vi "HPRF File Producer.vi"(3 "Source File":path=path "C:/ScopeBinaryData.bin", 4 "error in (no error)":errorcluster, 5 "# Channels":i32, 6 "Samples per Channel":i32, 7 "Data Queue":refnum<queue>) -> (0 "error out":errorcluster)   [LabVIEW 2013]
uses:
  ExecutionControlGlobal.vi
panel:
  out "Data":dbl[][](graph)
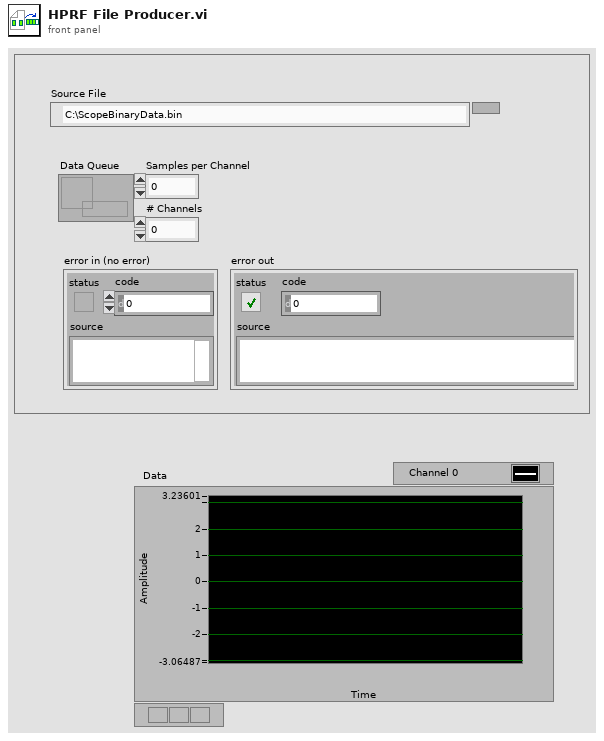
[diagram p1: front panel]
types:
  T1 = enum16{"open", "replace", "create", "open or create", "replace or create", "replace or create with confirmation"}
  T2 = enum16{"big-endian, network order", "native, host order", "little-endian"}
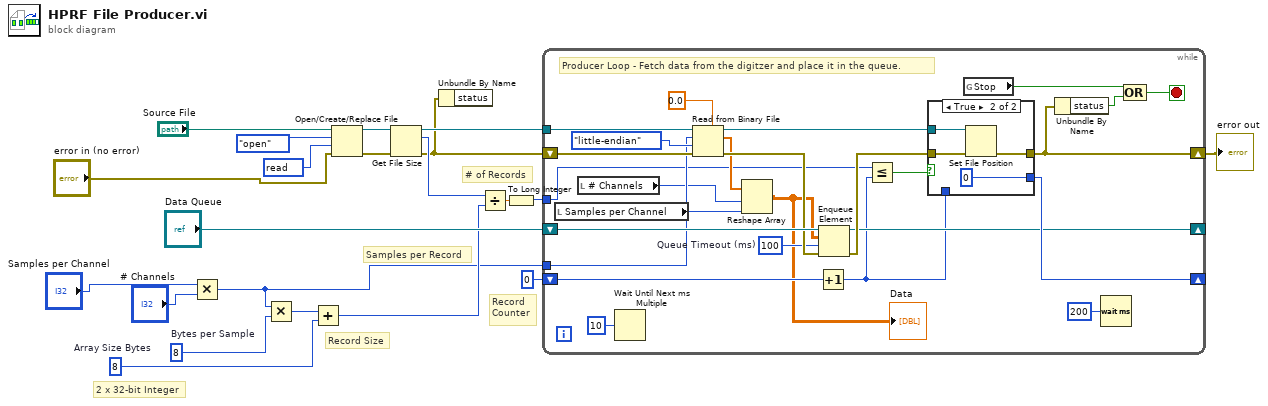
[diagram p0: block diagram]
diagram:
  w13 = 8  # Array Size Bytes
  w2 = 8  # Bytes per Sample
  w6 = u32 2147483648 items=["read"=2147483648, "write"=1073741824, "read & write"=3221225472, "execute"=536870912, "all"=268435456] ("desired access (read & write)")
  # "Samples per Record"
  # "# of Records"
  # "Record\nCounter"
  # "Record Size"
  # "2 x 32-bit Integer"
  n1 = Multiply(x="Samples per Channel", y="# Channels") -> (x*y=w1:i32)
  n2 = Multiply(x=w1, y=w2) -> (x*y=w3:i32)
  n3 = Add(x=w3, y=w13) -> (x+y=w12:i32)
  n4 = Open/Create/Replace File(file path (use dialog)="Source File", error in="error in (no error)", operation (0:open)=T1."open", access (0:read/write)=w6) -> (refnum out=w9:refnum<file>, error out=w10:errorcluster)  [unwired: 2 in, 1 out]
  n5 = Get File Size(file=w9, error in=w10) -> (refnum out=w21:refnum<file>, size (in bytes)=w20:i64, 0:w4:errorcluster)
  n6 = Unbundle By Name(w4) -> ()  [unwired: 1 out]
  n7 = Divide(x=w20, y=w12) -> (x/y=w19:dbl)
  n8 = To Long Integer(number=w19) -> (32bit integer=w18:i32)
  n9 = while {
    shift-right: [w43] -> w16
    shift-left: w4 -> [w44]
    tunnel: w21 -> [w45]
    shift-right: [w41] -> _
    shift-left: 0 -> [w31]
    tunnel: w18 -> [w25]
    shift-right: [w37] -> _
    shift-left: "Data Queue" -> [w40]
    tunnel: w1 -> [w27]
    stop <- w36 stop-if-true
    w34 = 100  # Queue Timeout (ms)
    # "Producer Loop - Fetch data from the digitzer and place it in the queue."
    n10 = local read "Samples per Channel"() -> (w23:i32)
    n11 = local read "# Channels"() -> (w24:i32)
    n12 = Wait Until Next ms Multiple(millisecond multiple=u32 10) -> ()  [unwired: 1 out]
    n13 = Read from Binary File(5:0.0, 8:w44, 9:T2."little-endian" ("byte order (0:big-endian, network order)"), 10:w27, 11:w45) -> (0:w39:errorcluster, 2:w26:dbl[], 3:w42:refnum<file>)  [unwired: 1 in, 1 out]
    n14 = Reshape Array(w26, w24, w23) -> (w22:dbl[][])
    "Data" <- w22
    n15 = Increment(x=w31) -> (x+1=w30:i32)
    n16 = Enqueue Element(queue=w40, element=w22, timeout in ms (-1)=w34, error in (no error)=w39) -> (queue out=w37:refnum<queue>, error out=w38:errorcluster)  [unwired: 1 out]
    n17 = Less Or Equal?(x=w25, y=w30) -> (x <= y?=w32:bool)
    n18 = case shown="True" w32 {
      tunnel: w38 -> [w49 w53]
      tunnel: [w49 w52] -> w43
      tunnel: w42 -> [_ w51]
      tunnel: [w48 0] -> w41
      tunnel: w30 -> [w48 _]
      frame False {
      }
      frame True {
        n19 = Set File Position(refnum=w51, error in=w53) -> (error out=w52:errorcluster)  [unwired: 2 in, 1 out]
      }
    }
    n20 = global read "ExecutionControlGlobal.vi" "Stop"() -> (w33:bool)
    n21 = Unbundle By Name(w43) -> ("status"=w46:bool)
    n22 = Wait (ms)(milliseconds to wait=u32 200) -> ()  [unwired: 1 out]
    n23 = Compound Arithmetic op=OR(w33, w46) -> (w36:bool)
  }
  "error out" <- w16
